vi "OCV DMM Configure Acquisition.vi"(7 "OCV DMM Range":dbl=10.0 min=0.0 max=0.0 step=1e-09 format="%#_8f", 8 "error in (no error)":errorcluster, 9 "OCV DMM Settling Time":dbl=0.0001 min=0.0 max=0.0 step=1e-09 format="%#_8f", 10 "OCV DMM Aperture Time":dbl=0.033 min=0.0 max=0.0 step=1e-09 format="%#_8f", 11 "Instrument Descriptor":refnum<k15>) -> (0 "error out":errorcluster, 3 "Refnum Out":refnum<k15>, 4 "Config Time":u32)   [LabVIEW 2019]
uses:
  <instrlib>/niDMM/nidmm.llb/niDMM Control Actions.ctl
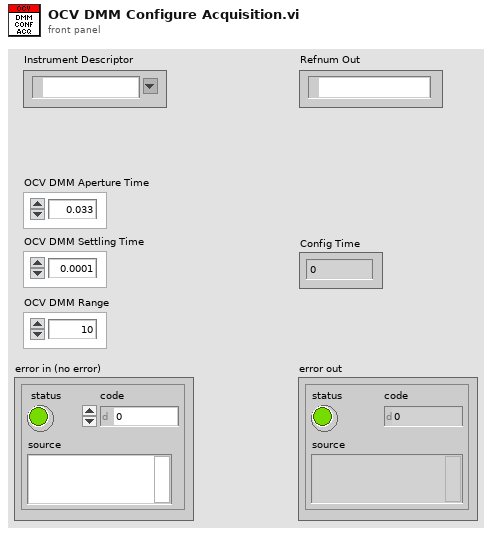
[diagram p1: front panel]
types:
  T1 = typedef "niDMM Control Actions.ctl" = i32
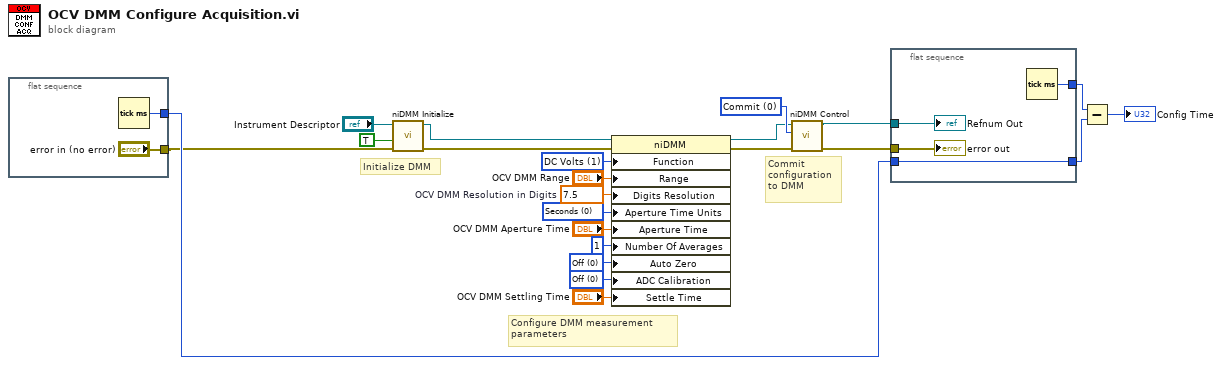
[diagram p0: block diagram]
diagram:
  w7 = 7.5 items=["3 1/2"=3.5, "4 1/2"=4.5, "5 1/2"=5.5, "6 1/2"=6.5, "7 1/2"=7.5]  # OCV DMM Resolution in Digits
  w10 = 1 items=["DC Volts"=1, "AC Volts"=2, "DC Current"=3, "AC Current"=4, "2-Wire Resistance"=5, "4-Wire Resistance"=101, "Frequency"=104, "Period"=105, "AC Volts DC Coupled"=1001, "Diode"=1002, "Waveform Voltage"=1003, "Waveform Current"=1004, "Capacitance"=1005, "Inductance"=1006, "Temperature"=108] ("Configuration:Function")
  w19 = 0 items=["Auto"=-1, "Off"=0, "On"=1] ("Configuration:Measurement Options:ADC Calibration")
  w18 = 0 items=["Auto"=-1, "Off"=0, "On"=1, "Once"=2] ("Configuration:Measurement Options:Auto Zero")
  w9 = 0 items=["Seconds", "Power Line Cycles"] ("Configuration:Advanced:Aperture Time Units")
  w16 = T1 0 items=["Commit"] ("Control Action")
  # "Commit\nconfiguration\nto DMM"
  # "Configure DMM measurement \nparameters"
  # "Initialize DMM"
  n1 = flat-sequence {
    tunnel: [w25] -> w23
    tunnel: ["error in (no error)"] -> w2
    frame #0 {
      n2 = Tick Count (ms)() -> (millisecond timer value=w25:u32)
    }
  }
  n3 = call <instrlib>:"niDMM Initialize.vi"("error in (no error)"=w2, "Reset"=TRUE, "Instrument Descriptor"="Instrument Descriptor") -> ("error out"=w12:errorcluster, "instrument handle out"=w11:refnum<k15>)  [unwired: 7 in]
  n4 = property class="niDMM"(reference=w11, error in=w12, "Function"=w10, "Range"="OCV DMM Range", "Digits Resolution"=w7, "Aperture Time Units"=w9, "Aperture Time"="OCV DMM Aperture Time", "Number Of Averages"=1 ("Configuration:Advanced:Number Of Averages"), "Auto Zero"=w18, "ADC Calibration"=w19, "Settle Time"="OCV DMM Settling Time") -> (reference out=w14:refnum<k15>, error out=w15:errorcluster)
  n5 = call <instrlib>:"niDMM Control.vi"("error in (no error)"=w15, "Control Action"=w16, "instrument handle"=w14) -> ("error out"=w3:errorcluster, "instrument handle out"=w4:refnum<k15>)  [unwired: 7 in]
  n6 = flat-sequence {
    tunnel: [w29] -> w22
    tunnel: w4 -> [w26]
    tunnel: w3 -> [w28]
    tunnel: w23 -> [w27]
    tunnel: [w27] -> w21
    frame #0 {
      n7 = Tick Count (ms)() -> (millisecond timer value=w29:u32)
      "error out" <- w28
      "Refnum Out" <- w26
    }
  }
  n8 = Subtract(x=w22, y=w21) -> (x-y=→"Config Time":u32)
